vi "stop.vi"(8 "error in (no error)":errorcluster) -> (0 "error out":errorcluster)   [LabVIEW 2017, in "libfreenect.lvlib"]
doc: "EXPORT void freenect_lv_stop();"
uses:
  libfreenect.lvlib
  freenect_lv.dll
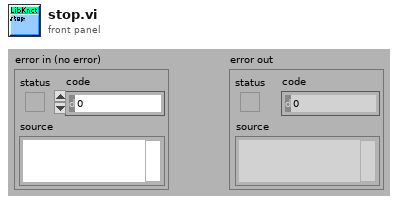
[diagram p1: front panel]
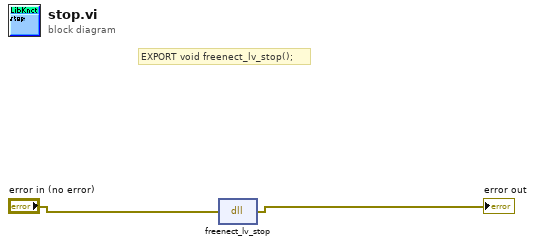
[diagram p0: block diagram]
diagram:
  # "EXPORT void freenect_lv_stop();"
  n1 = dll-call lib="C:/Users/Mats/Desktop/Bacheler prosjekt/Labview/Occupancy Grid Map Code - With model/freenect_lv.*" fn="freenect_lv_stop"(error in="error in (no error)") -> (error out=→"error out":errorcluster)  [unwired: 2 in, 2 out]
